vi "Ohaus AV Series Continuous Measurement.vi"() -> ()   [LabVIEW 2015]
doc: "This VI initializes the balance with default settings and continuously takes the weight measurement without waiting for stabilize until user presses the stop button. The actual weight is displayed in numeric indicator and chart graph.\n\n<B>Before running this VI some initial instrument setup is required:</B>\nOnly Gross, Net, Tare; Reference; and GLP need to be changed from their default values to OFF\n\nGoto the menu screen on the balance\n Then the PRINT-1 menu\n \n Output\n When Stable: OFF (default) \n GLP Tare: OFF (default)\n Auto Print: OFF (default)\n Content\n Number Only: OFF (default)\n Header: OFF (default)\n<B> Gross, Net, and Tare: OFF</B>\n<B> Reference: OFF</B>\n Result: ON (default)\n<B> GLP: OFF</B>\n Layout\n Line Format: MULTI (default)\n Line Feed: OFF (default)\n Form Feed: OFF (default)"
uses:
  Ohaus AV Series.lvlib
panel:
  in  "Serial Configuration":T1={"Baud Rate (2400)"=2400, "Flow Control (1: XON/XOFF)"=1, "Parity (0: None)"=0, "Data Bits (7)"=7} {"Data Bits (7)" items=["7"=7, "8"=8]; "Parity (0: None)" items=["None", "Odd", "Even"]; "Flow Control (1: XON/XOFF)" items=["None", "XON/XOFF", "RTS/CTS"]; "Baud Rate (2400)" items=["600"=600, "1200"=1200, "2400"=2400, "4800"=4800, "9600"=9600, "19200"=19200]}
  in  "VISA resource name":refnum<visa-resource-name>
  in  "Units (0: Gram)":u16(ring) items=["Gram (g)"=0, "Kilogram (kg)"=1, "Penny weight (dwt)"=2, "Carat (ct)"=3, "Ounce (oz)"=4, "Ounce Troy (oz t)"=5, "Grain (GN)"=6, "Hong Kong Tael (HKt)"=7, "Singapore Tael (SGt)"=8, "Tiwan Tael (TWt)"=9, "Momme (m)"=10, "Pound (lb)"=11, "Newton (N)"=13, "Tical (ti)"=14, "Tula"=15, "Mesghal (Meshg)"=16, "Baht"=17, "Custom"=19]
  in  "Stop":bool
  out "Waveform Chart":dbl(graph)
  out "Current Weight Value":dbl format="%.2p"
  # "(c) 2004-2009 National Instruments.  All Rights Reserved."
  # "OHAUS Adventurer Pro"
  # "Before running this VI some initial setup is required\n(See VI documentation for more information)"
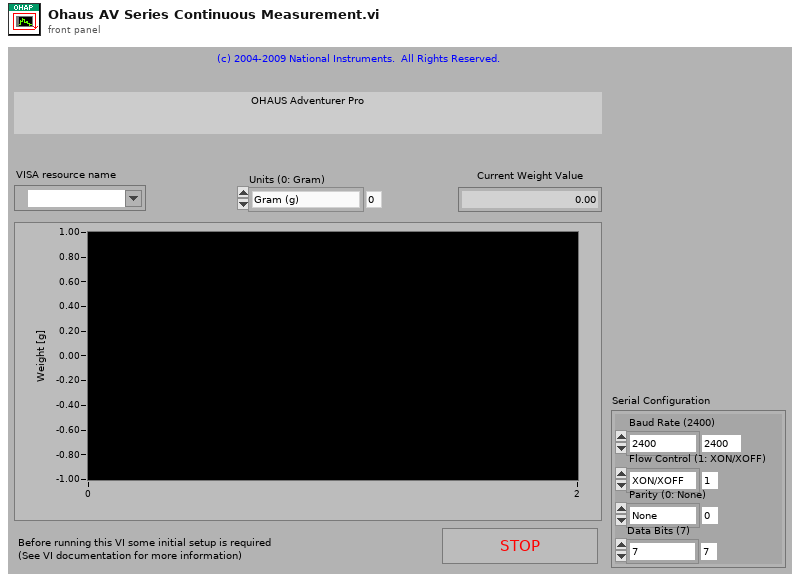
[diagram p1: front panel]
types:
  T1 = cluster{"Baud Rate (2400)":u32, "Flow Control (1: XON/XOFF)":u16, "Parity (0: None)":u16, "Data Bits (7)":u16}
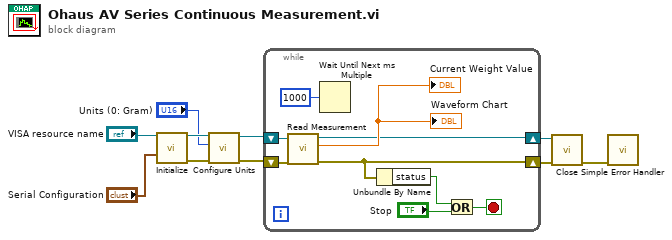
[diagram p0: block diagram]
diagram:
  n1 = call "Initialize.vi"("VISA resource name"="VISA resource name", "Serial Configuration"="Serial Configuration") -> ("VISA resource name out"=w6:refnum<visa-resource-name>, "error out"=w5:errorcluster)  [unwired: 12 in]
  n2 = call "Configure Units.vi"("error in (no error)"=w5, "Units (0: Gram)"="Units (0: Gram)", "VISA resource name"=w6) -> ("error out"=w4:errorcluster, "VISA resource name out"=w7:refnum<visa-resource-name>)  [unwired: 7 in]
  n3 = while {
    shift-right: [w14] -> w9
    shift-left: w4 -> [w16]
    shift-right: [w15] -> w10
    shift-left: w7 -> [w17]
    stop <- w12 stop-if-true
    n4 = call "Read Measurement.vi"("error in (no error)"=w16, "VISA resource name"=w17) -> ("error out"=w14:errorcluster, "Weight Value"=→"Current Weight Value" →"Waveform Chart":dbl, "VISA resource name out"=w15:refnum<visa-resource-name>)  [unwired: 4 in, 3 out]
    n5 = Wait Until Next ms Multiple(millisecond multiple=u32 1000 ("milliseconds to wait")) -> ()  [unwired: 1 out]
    n6 = Unbundle By Name(w14) -> ("status"=w13:bool)
    n7 = Or(x=w13, y="Stop") -> (x .or. y?=w12:bool)
  }
  n8 = call "Close.vi"("error in (no error)"=w9, "VISA resource name"=w10) -> ("error out"=w8:errorcluster)  [unwired: 9 in]
  n9 = call <vilib>:"Simple Error Handler.vi"("error in (no error)"=w8) -> ()  [unwired: 4 in, 5 out]
